vi "InitFreqFiles.vi"(8 "error in":errorcluster, 10 "FileName":string="72.txt") -> (0 "error out":errorcluster, 2 "value":dbl, 3 "path":path)   [LabVIEW 2018]
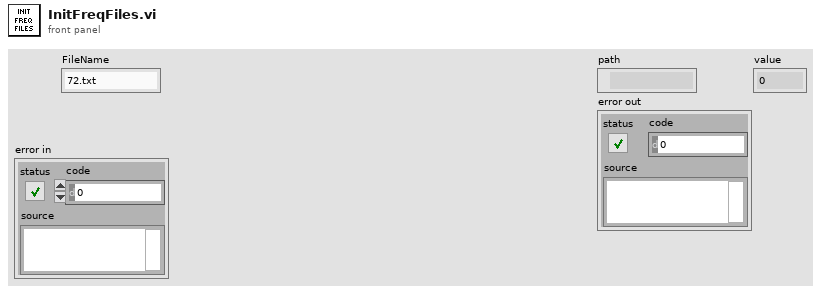
[diagram p1: front panel]
types:
  T1 = enum16{"open", "replace", "create", "open or create", "replace or create", "replace or create with confirmation"}
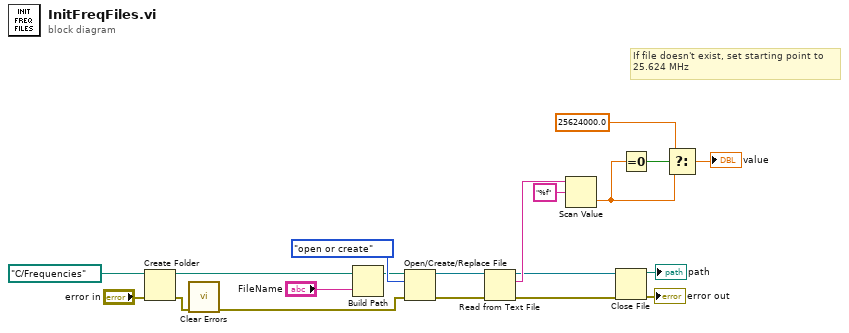
[diagram p0: block diagram]
diagram:
  # "If file doesn't exist, set starting point to \n25.624 MHz"
  n1 = Create Folder(path (use dialog)=path "C:/Frequencies", error in="error in") -> (created path=w18:path, error out=w16:errorcluster)  [unwired: 1 in, 1 out]
  n2 = call <vilib>:"Clear Errors.vi"("error in (no error)"=w16) -> ("error out"=w15:errorcluster)  [unwired: 5 in, 1 out]
  n3 = Build Path(base path=w18, name or relative path="FileName") -> (appended path=w10:path)
  n4 = Open/Create/Replace File(file path (use dialog)=w10, error in=w15, operation (0:open)=T1."open or create") -> (refnum out=w17:refnum<file>, error out=w20:errorcluster)  [unwired: 3 in, 1 out]
  n5 = Read from Text File(file (use dialog)=w17, error in=w20) -> (refnum out=w12:refnum<file>, text=w19:string, error out=w13:errorcluster)  [unwired: 2 in, 1 out]
  n6 = Scan Value(string=w19, format string="%f") -> (value=w4:dbl)  [unwired: 1 in, 1 out]
  n7 = Close File(refnum=w12, error in=w13) -> (path=→"path":path, error out=→"error out":errorcluster)
  n8 = Equal To 0?(x=w4) -> (x = 0?=w5:bool)
  n9 = Select(t=25624000.0 ("ManualFreq"), s=w5, f=w4) -> (s? t:f=→"value":dbl)
